vi "Measurement UI.vi"() -> ()   [LabVIEW 2023]
panel:
  out "Measure record dt":dbl
  in  "MeasGraphs":T1(tab)
  out "EfficiencyGraph":T2(graph)
  out "LoadRegulationGraph(V/A)":T3(graph)
  out "LoadRegulationGraph(%)":T3(graph)
  out "OutputCurrentV/STimeGraph":waveform(dbl)(graph) caption="Load Transient"
  in  "Load Current v/s Time":string="LOAD CURRENT vs TIME"
  in  "Output Voltage v/s Time":string="LOAD VOLTAGE vs TIME"
  out "OutputVoltageV/STimeGraph":waveform(dbl)(graph) caption="Load Transient"
  out "Ganged load transient voltages":dbl[](array[numeric])
  out "Ganged load transient currents":dbl[](array[numeric])
  out "Load voltage deviation":dbl[](array[numeric])
  out "Ganged load voltages":dbl[](array[numeric])
  in  "Load current pole-zero ratio":dbl=0.3
  in  "Load current compensation frequency":dbl=180000.0
  in  "Load current gain bandwidth":dbl=14000.0
  in  "Source voltage pole-zero ratio":dbl=2.0
  in  "Source voltage compensation frequency":dbl=3530.0
  in  "Source voltage gain bandwidth":dbl=2000.0
  in  "Load slave resource names":string[](array[string])
  in  "Load master resource name":string
  in  "Source slave resource names":string[](array[string])
  in  "Source master resource name":string
  out "Load sweep points":i32
  out "Source sweep points":i32
  out "Voltage values":dbl[](array[numeric])
  out "Efficiency":dbl[](array[numeric])
  out "Ganged load currents":dbl[](array[numeric])
  in  "MeasConfigurations":T4(tab)=enum."Source Config"
  in  "Measurement timeout":dbl=10.0 caption="MEASUREMENT TIME-OUT" format="%.3ps"
  in  "Nominal output voltage":dbl=1.0 caption="NOMINAL OUTPUT VOLTAGE" format="%.3fV"
  in  "Source delay":dbl=0.005 caption="SOURCE DELAY" format="%.3ps"
  in  "DUT setup time":dbl=1.0 caption="DUT SETUP TIME" format="%.3ps"
  in  "Aperture time":dbl=0.005 caption="APERTURE TIME" format="%.3ps"
  in  "PPSSlaveResourceNames":refnum<k15>[](array[refnum]) caption="SLAVE RESOURCE NAMES"
  in  "PPSMasterResourceName":refnum<k15> caption="MASTER RESOURCE NAME"
  in  "Source stop voltage":dbl=14.0 caption="VOLTAGE STOP LEVEL" format="%#_6pV"
  in  "Source transient response":i32(ring)=1038 caption="TRANSIENT RESPONSE" items=["Slow"=1041, "Normal"=1038, "Fast"=1039, "Custom"=1042]
  in  "Source sense":i32(ring)=1009 caption="SENSE" items=["Local"=1008, "Remote"=1009]
  in  "Source voltage level range":dbl=20.0 caption="VOLTAGE LEVEL RANGE" format="%#_6pV"
  in  "Source start voltage":dbl=6.0 caption="VOLTAGE START LEVEL" format="%#_6pV"
  in  "Source current limit high":dbl=25.0 caption="CURRENT LIMIT/LIMIT HIGH" format="%#_6pA"
  in  "Source current limit range":dbl=25.0 caption="CURRENT LIMIT RANGE" format="%#_6pA"
  in  "Source limit symmetry":enum32{"Symmetric", "Asymmetric"}(ring)=enum."Asymmetric" caption="LIMIT SYMMETRY"
  in  "Source current limit low":dbl=-0.6 caption="CURRENT LIMIT LOW" format="%#_6pA"
  in  "Source system configuration":enum32{"Series", "Parallel"}(ring)=enum."Parallel" caption="SYSTEM CONFIG"
  in  "Source compliance":string="Compliance"
  in  "Source sourceadapt":string="SourceAdapt"
  in  "Source voltage sweep points":i32=4 caption="NO. OF POINTS"
  in  "Source Custom Transient Response":bool
  in  "Load current sweep points/points per decade":i32=10 caption="PTS/PTS PER DECADE"
  in  "Load sweep type":string(combo)="Logarithmic" caption="SWEEP TYPE"
  in  "Load stop current":dbl=50.0 caption="CURRENT STOP LEVEL" format="%#_6pA"
  in  "Load sourceadapt":string="SourceAdapt"
  in  "Load compliance":string="Compliance"
  in  "Load system configuration":enum32{"Series", "Parallel"}(ring)=enum."Parallel" caption="SYSTEM CONFIG"
  in  "Load voltage limit low":dbl caption="VOLTAGE  LIMIT LOW" format="%#_6pV"
  in  "Load limit symmetry":enum32{"Symmetric", "Asymmetric"}(ring) caption="LIMIT SYMMETRY"
  in  "Load voltage limit range":dbl=6.0 caption="VOLTAGE LIMIT RANGE" format="%#_6pV"
  in  "Load voltage limit high":dbl=inf caption="VOLTAGE LIMIT/LIMIT HIGH" format="%#_6p"
  in  "Load start current":dbl=2.0 caption="CURRENT START LEVEL" format="%#_6pA"
  in  "Load current level range":dbl=80.0 caption="CURRENT LEVEL RANGE" format="%#_6pA"
  in  "Load sense":i32(ring)=1009 caption="SENSE" items=["Local"=1008, "Remote"=1009]
  in  "Load transient response":i32(ring)=1038 caption="TRANSIENT RESPONSE" items=["Slow"=1041, "Normal"=1038, "Fast"=1039, "Custom"=1042]
  in  "LoadSlaveResourceNames":refnum<k15>[](array[refnum]) caption="SLAVE RESOURCE NAMES"
  in  "LoadMasterResourceName":refnum<k15> caption="MASTER RESOURCE NAME"
  in  "Load Custom Transient Response":bool
  in  "Sample rate":dbl=0.001 caption="SAMPLE RATE" format="%.3pS/s"
  in  "Level dwell time":dbl=0.001 caption="DWELL TIME" format="%.3ps"
  in  "Enable load transient test?":bool
  in  "Load current falling slew rate":dbl=24.0 caption="CURRENT FALLING SLEW RATE" format="%#_6pA/us"
  in  "Load current rising slew rate":dbl=24.0 caption="CURRENT RISING SLEW RATE" format="%#_6pA/us"
  in  "Load current set point 2":dbl=20.0 caption="CURRENT SET POINT 2" format="%#_6pA"
  in  "Load current set point 1":dbl=1.0 caption="CURRENT SET POINT 1" format="%#_6pA"
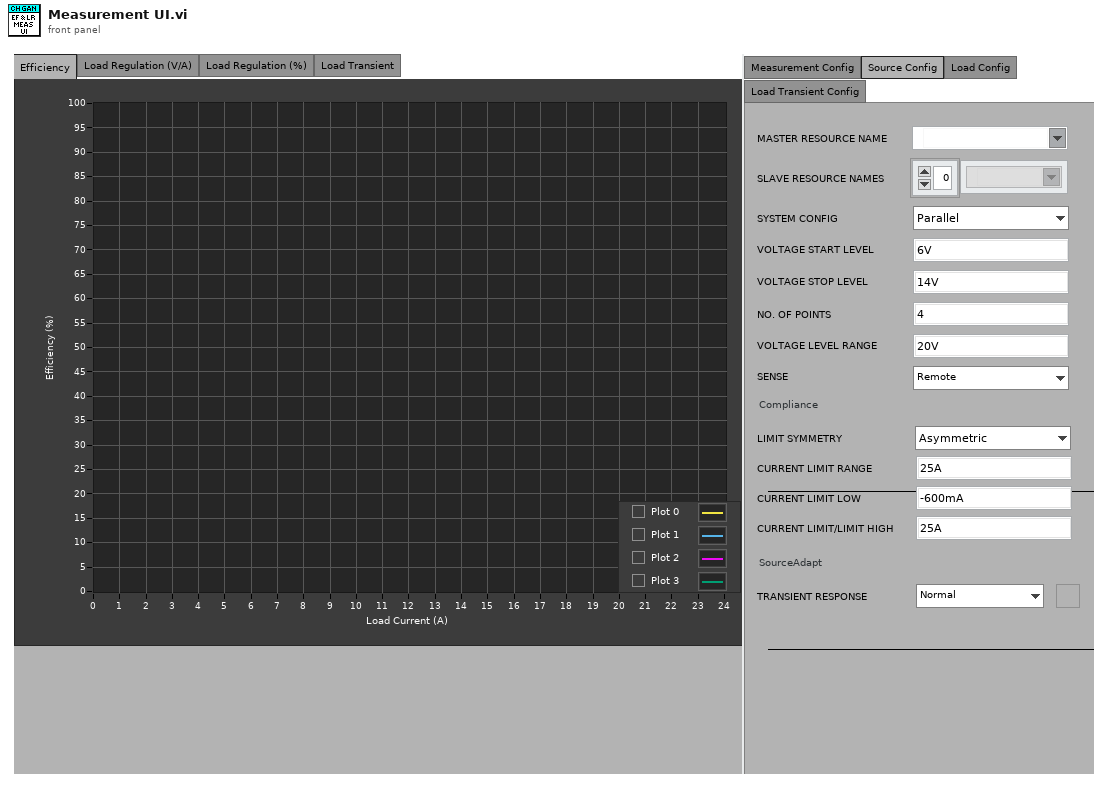
[diagram p1: front panel]
types:
  T1 = enum32{"Efficiency", "Load Regulation (V/A)", "Load Regulation (%)", "Load Transient", "Hidden Controls"}
  T2 = cluster{"Ganged load currents":dbl[], "Efficiency":dbl[]}[]
  T3 = cluster{"Load currents":dbl[], "Efficiency":dbl[]}[]
  T4 = enum32{"Measurement Config", "Source Config", "Load Config", "Load Transient Config"}
  T5 = typedef "SourceAdapt Parameters.ctl" = cluster{"Voltage gain bandwidth":dbl, "Voltage compensation frequency":dbl, "Voltage pole-zero ratio":dbl, "Current gain bandwidth":dbl, "Current compensation frequency":dbl, "Current pole-zero ratio":dbl}
  T6 = cluster{"Ganged load currents":dbl[], "Efficiency":dbl[]}
  T7 = cluster{"Ganged load currents":dbl[], "Ganged load voltages":dbl[]}
  T8 = cluster{"Ganged load currents":dbl[], "Load voltage deviation":dbl[]}
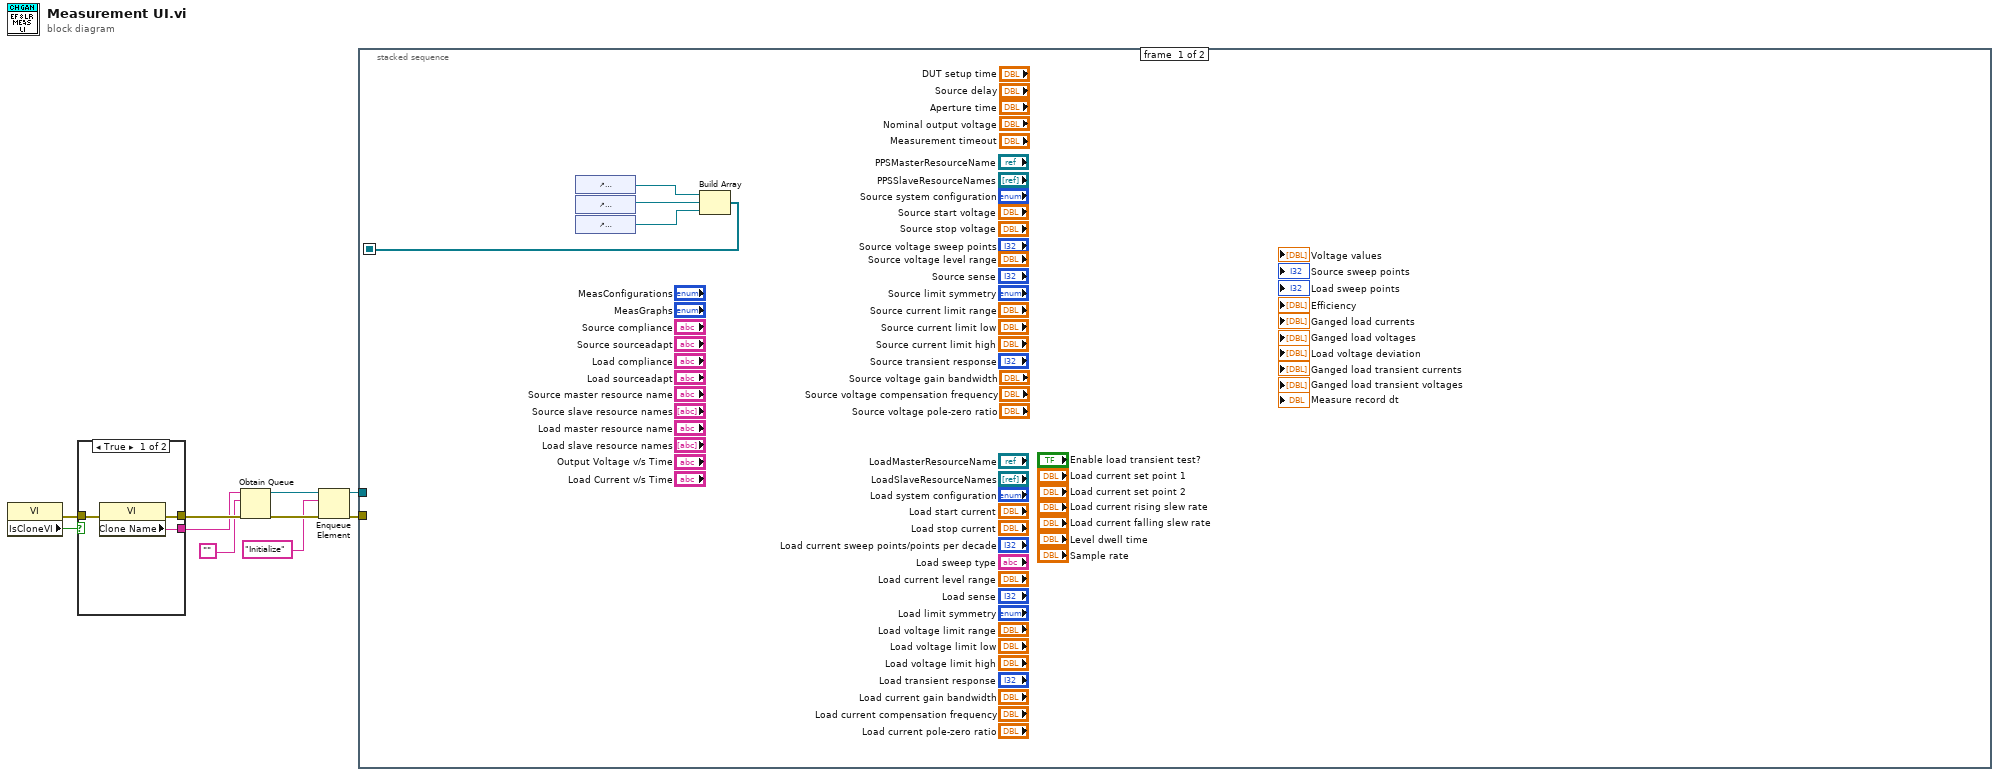
[diagram p0: block diagram]
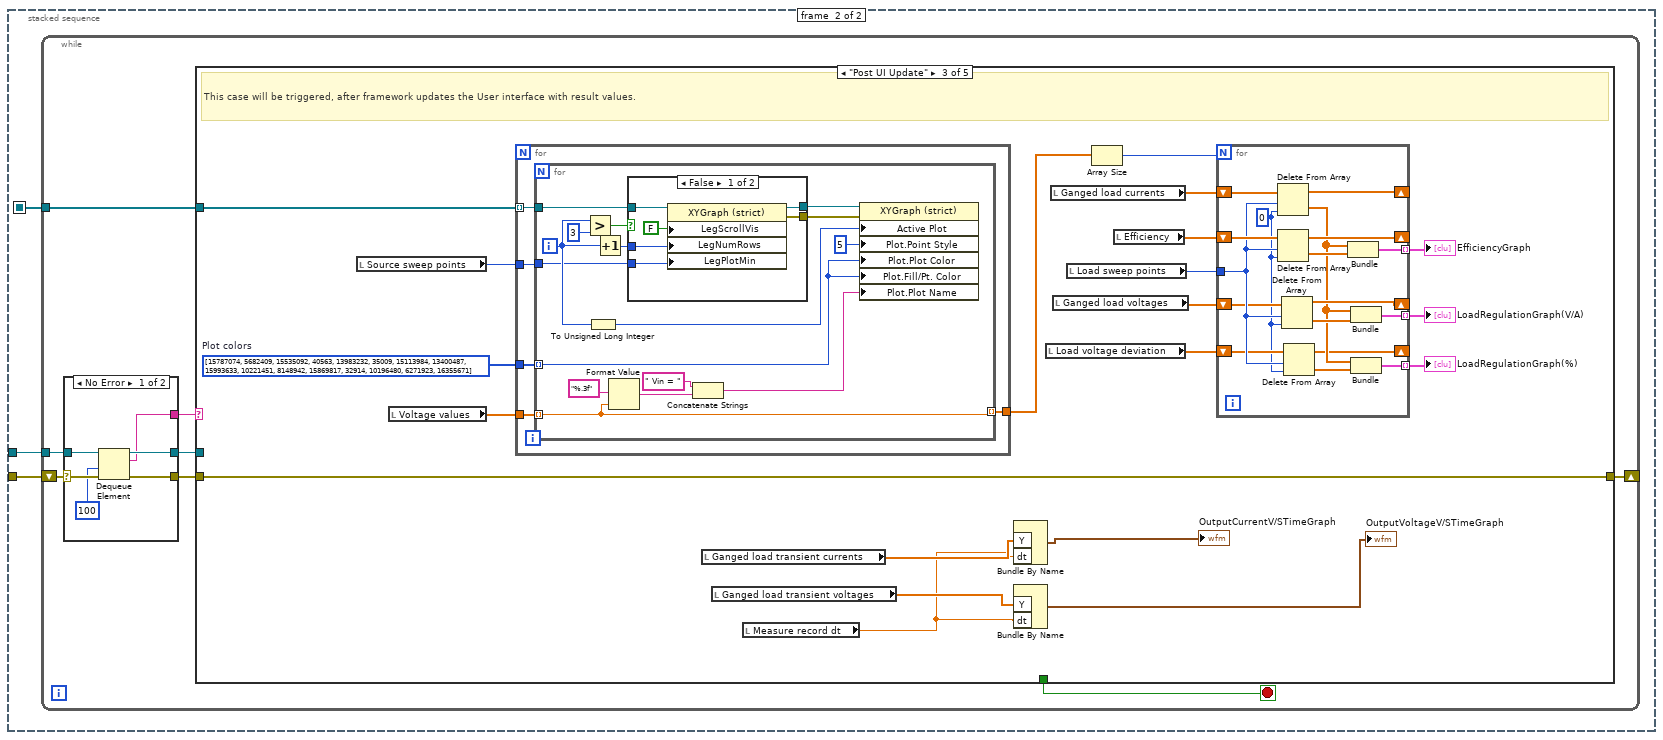
[diagram p2: hidden frame]
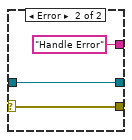
[diagram p3: hidden frame]
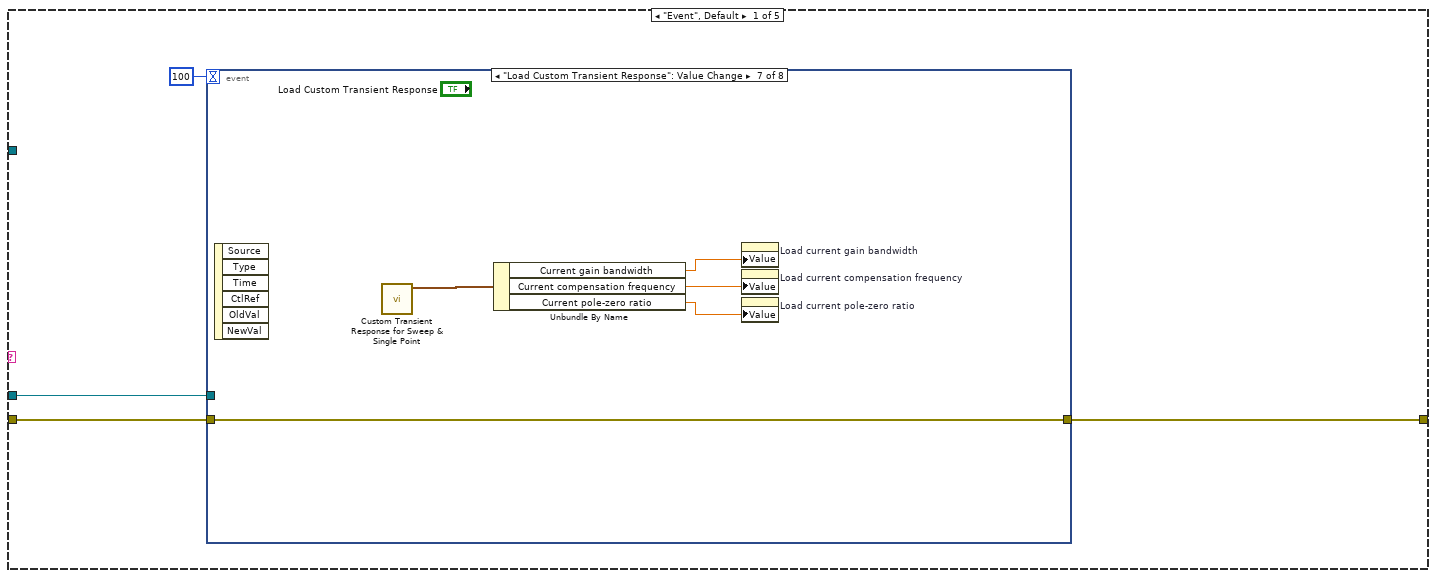
[diagram p4: hidden frame]
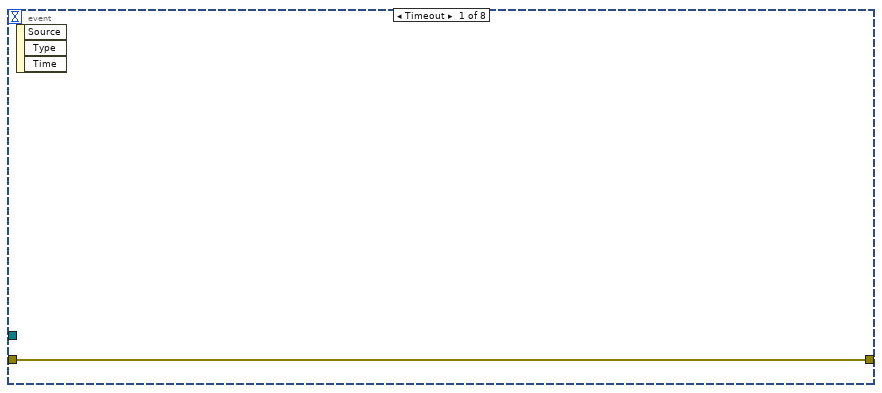
[diagram p5: hidden frame]
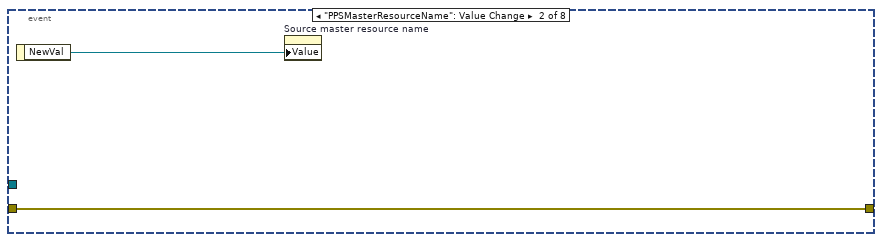
[diagram p6: hidden frame]
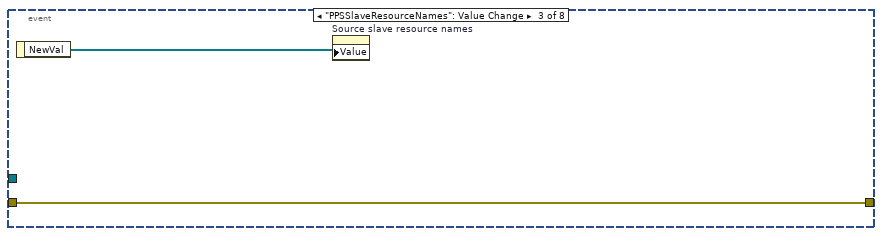
[diagram p7: hidden frame]
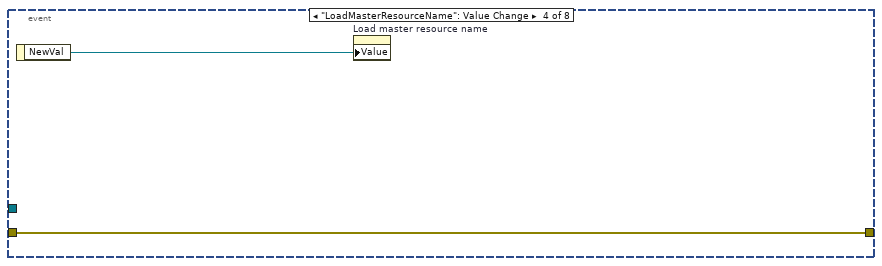
[diagram p8: hidden frame]
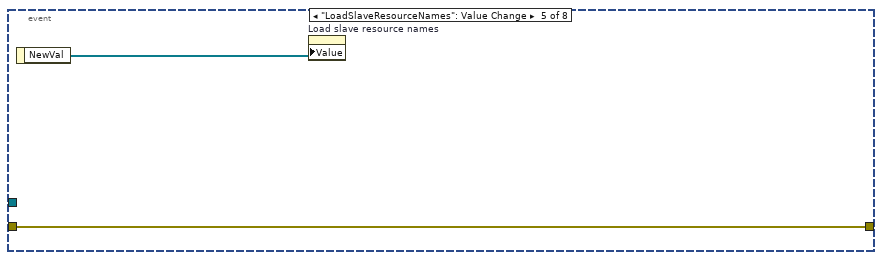
[diagram p9: hidden frame]
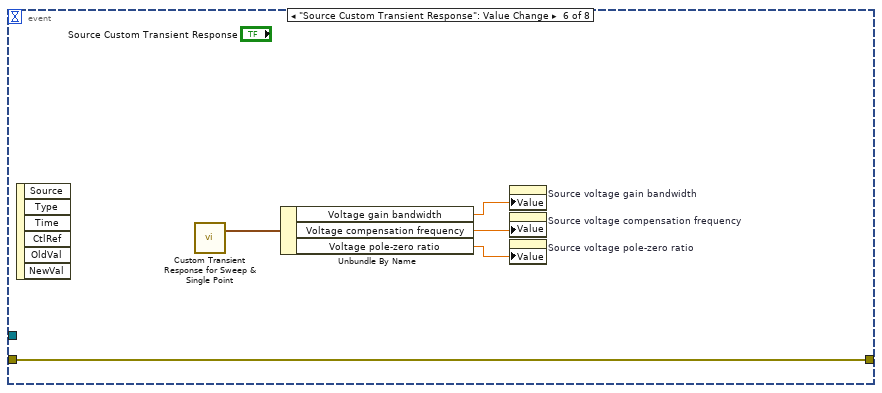
[diagram p10: hidden frame]
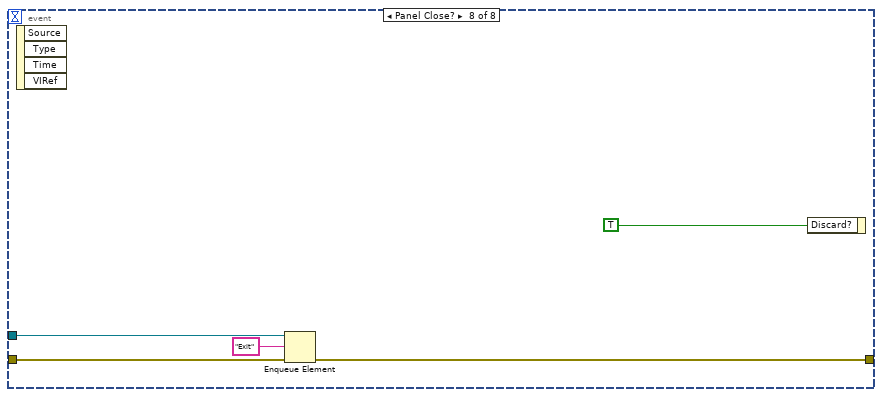
[diagram p11: hidden frame]
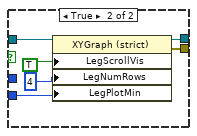
[diagram p13: hidden frame]
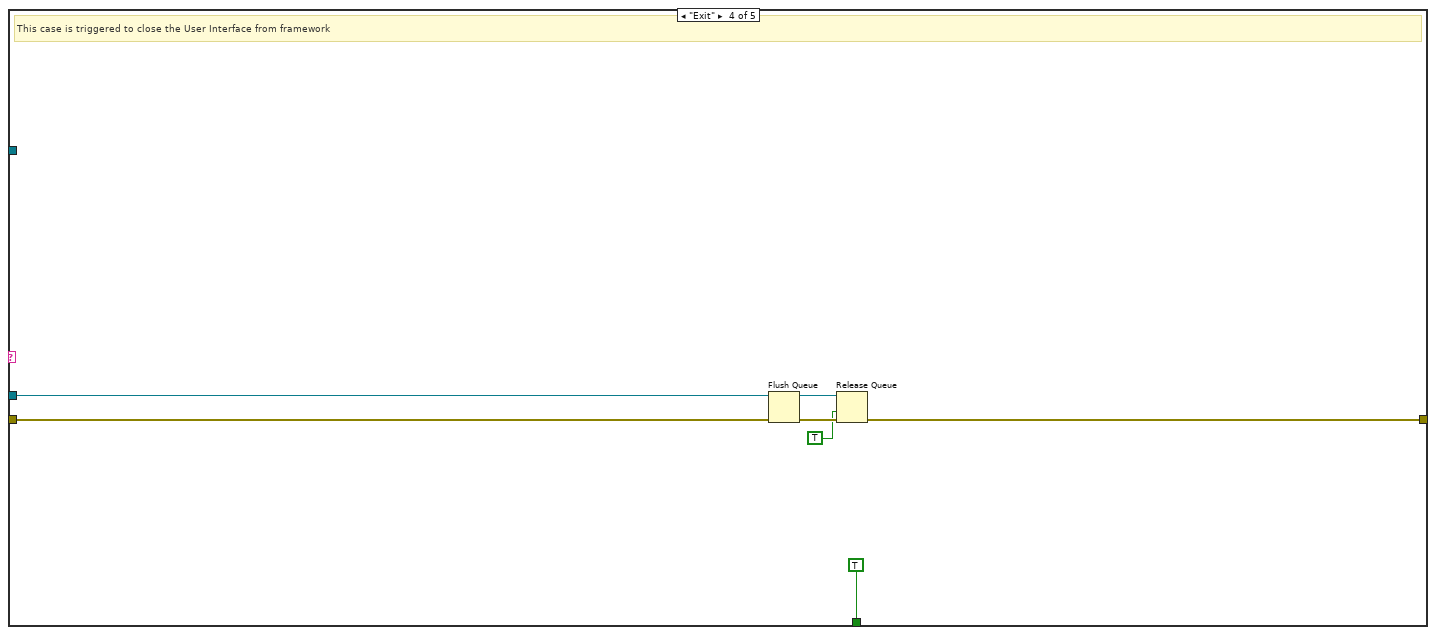
[diagram p14: hidden frame]
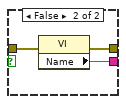
[diagram p16: hidden frame]
diagram:
  n1 = property class="VI"() -> (error out=w1:errorcluster, "IsCloneVI"=w2:bool)  [unwired: 2 in, 1 out]
  n2 = case shown="True" w2 {
    tunnel: [w13 w16] -> w10
    tunnel: [w12 w15] -> w9
    tunnel: w1 -> [w11 w14]
    frame True {
      n3 = property class="VI"(error in=w11) -> (error out=w13:errorcluster, "Clone Name"=w12:string)  [unwired: 1 in, 1 out]
    }
    frame False {
      n4 = property class="VI"(error in=w14) -> (error out=w16:errorcluster, "Name"=w15:string)  [unwired: 1 in, 1 out]
    }
  }
  n5 = Obtain Queue(name (unnamed)=w9, element data type="", error in (no error)=w10) -> (queue out=w6:refnum<queue>, error out=w8:errorcluster)  [unwired: 2 in, 1 out]
  n6 = Enqueue Element(queue=w6, element="Initialize", error in (no error)=w8) -> (queue out=w5:refnum<queue>, error out=w7:errorcluster)  [unwired: 1 in, 1 out]
  n7 = stacked-sequence {
    seq-local: [w17 _] -> [_ w21]
    tunnel: w7 -> [_ w23]
    tunnel: w5 -> [_ w22]
    frame #0 {
      n8 = control-ref of="EfficiencyGraph"() -> (w20:refnum<vi>)
      n9 = control-ref of="LoadRegulationGraph(V/A)"() -> (w19:refnum<vi>)
      n10 = control-ref of="LoadRegulationGraph(%)"() -> (w18:refnum<vi>)
      n11 = Build Array(w20, w19, w18) -> (w17:refnum<vi>[])
    }
    frame #1 {
      n12 = while {
        shift-right: [w26] -> _
        shift-left: w23 -> [w31]
        tunnel: w22 -> [w29]
        tunnel: w21 -> [w24]
        stop <- w25 stop-if-true
        n13 = case shown="No Error" w31 {
          selector: w31 -> [w37 w40]
          tunnel: [w36 w40] -> w30
          tunnel: w29 -> [w35 w39]
          tunnel: [w34 w39] -> w28
          tunnel: [w33 "Handle Error"] -> w27
          frame No Error {
            n14 = Dequeue Element(queue=w35, timeout in ms (-1)=100, error in (no error)=w37) -> (queue out=w34:refnum<queue>, element=w33:string, error out=w36:errorcluster)  [unwired: 1 out]
          }
          frame Error {
          }
        }
        n15 = case shown="\"Post UI Update\"" w27 {
          tunnel: w30 -> [w43 w69 w89 w146 w147]
          tunnel: w28 -> [w41 _ _ w144 _]
          tunnel: [w44 w69 w89 w141 w147] -> w26
          tunnel: [_ _ _ TRUE _] -> w25
          tunnel: w24 -> [_ _ w77 _ _]
          frame "Event", Default {
            n16 = event shown="[6] \"Load Custom Transient Response\": Value Change" {
              selector: _ -> [_ _ _ _ _ _ _ _]
              dyn-events: _ -> [_ _ _ _ _ _ _ _]
              timeout: 100 -> [_ _ _ _ _ _ _ _]
              tunnel: [w45 w47 w49 w50 w52 w57 w62 w66] -> w44
              tunnel: w43 -> [w45 w47 w49 w50 w52 w57 w62 w67]
              tunnel: w41 -> [_ _ _ _ _ _ _ w65]
              event Timeout {
                n17 = event-data() -> ()  [unwired: 1 in, 3 out]
              }
              event "PPSMasterResourceName": Value Change {
                n18 = event-data() -> ("NewVal"=w46:refnum<k15>)  [unwired: 1 in]
                n19 = property on="Source master resource name" class="Str"("Value"=w46) -> ()  [unwired: 2 in, 2 out]
              }
              event "PPSSlaveResourceNames": Value Change {
                n20 = event-data() -> ("NewVal"=w48:refnum<k15>[])  [unwired: 1 in]
                n21 = property on="Source slave resource names" class="Arr (strict)"("Value"=w48) -> ()  [unwired: 2 in, 2 out]
              }
              event "LoadMasterResourceName": Value Change {
                n22 = event-data() -> ("NewVal"=w51:refnum<k15>)  [unwired: 1 in]
                n23 = property on="Load master resource name" class="Str"("Value"=w51) -> ()  [unwired: 2 in, 2 out]
              }
              event "LoadSlaveResourceNames": Value Change {
                n24 = event-data() -> ("NewVal"=w53:refnum<k15>[])  [unwired: 1 in]
                n25 = property on="Load slave resource names" class="Arr (strict)"("Value"=w53) -> ()  [unwired: 2 in, 2 out]
              }
              event "Source Custom Transient Response": Value Change {
                n26 = event-data() -> ()  [unwired: 1 in, 6 out]
                n27 = call "Custom Transient Response for Sweep & Single Point.vi"() -> ("SourceAdapt Parameters"=w58:T5)  [unwired: 11 in]
                n28 = Unbundle By Name(w58) -> ("Voltage gain bandwidth"=w55:dbl, "Voltage compensation frequency"=w56:dbl, "Voltage pole-zero ratio"=w54:dbl)
                n29 = property on="Source voltage gain bandwidth" class="DigNum (strict)"("Value"=w55) -> ()  [unwired: 2 in, 2 out]
                n30 = property on="Source voltage compensation frequency" class="DigNum (strict)"("Value"=w56) -> ()  [unwired: 2 in, 2 out]
                n31 = property on="Source voltage pole-zero ratio" class="DigNum (strict)"("Value"=w54) -> ()  [unwired: 2 in, 2 out]
              }
              event "Load Custom Transient Response": Value Change {
                n32 = event-data() -> ()  [unwired: 1 in, 6 out]
                n33 = call "Custom Transient Response for Sweep & Single Point.vi"() -> ("SourceAdapt Parameters"=w63:T5)  [unwired: 11 in]
                n34 = Unbundle By Name(w63) -> ("Current gain bandwidth"=w59:dbl, "Current compensation frequency"=w61:dbl, "Current pole-zero ratio"=w60:dbl)
                n35 = property on="Load current gain bandwidth" class="DigNum (strict)"("Value"=w59) -> ()  [unwired: 2 in, 2 out]
                n36 = property on="Load current compensation frequency" class="DigNum (strict)"("Value"=w61) -> ()  [unwired: 2 in, 2 out]
                n37 = property on="Load current pole-zero ratio" class="DigNum (strict)"("Value"=w60) -> ()  [unwired: 2 in, 2 out]
              }
              event Panel Close? {
                n38 = event-data() -> ()  [unwired: 1 in, 4 out]
                n39 = Enqueue Element(queue=w65, element="Exit", error in (no error)=w67) -> (error out=w66:errorcluster)  [unwired: 1 in, 2 out]
                n40 = event-data("Discard?"=TRUE) -> ()  [unwired: 1 in, 1 out]
              }
            }
          }
          frame "Initialize" {
          }
          frame "Post UI Update" {
            w84 = u32[] [15787074, 5682409, 15535092, 40563, 13983232, 35009, 15113984, 13400487, 15993633, 10221451, 8148942, 15869817, 32914, 10196480, 6271923, 16355671]  # Plot colors
            # "This case will be triggered, after framework updates the User interface with result values."
            n41 = local read "Source sweep points"() -> (w82:i32)
            n42 = local read "Voltage values"() -> (w83:dbl[])
            n43 = for {
              tunnel: w84 -> [w94]
              tunnel: w77 -> [w93] mode=indexing
              tunnel: w83 -> [w92]
              tunnel: w82 -> [w91]
              tunnel: [w90] -> w76
              n44 = for {
                tunnel: w92 -> [w107] mode=indexing
                tunnel: [w107] -> w90 mode=indexing
                tunnel: w93 -> [w100]
                tunnel: w91 -> [w97]
                tunnel: w94 -> [w103] mode=indexing
                i -> [w101]
                n45 = Greater?(x=w101, y=3) -> (0:w105:bool)
                n46 = To Unsigned Long Integer(number=w101) -> (unsigned 32bit integer=w104:u32)
                n47 = Increment(x=w101) -> (x+1=w99:i32)
                n48 = Format Value(format string="%.3f", value (0)=w107) -> (output string=w110:string)  [unwired: 1 out]
                n49 = case shown="False" w105 {
                  tunnel: w100 -> [w116 w122]
                  tunnel: w99 -> [w115 _]
                  tunnel: [w114 w121] -> w98
                  tunnel: w97 -> [w112 w117]
                  tunnel: [w113 w120] -> w96
                  frame False {
                    n50 = property on="Property Node" class="XYGraph (strict)"(reference=w116, "LegScrollVis"=FALSE ("Legend:Scrollbar Visible"), "LegNumRows"=w115, "LegPlotMin"=w112) -> (reference out=w114:refnum<vi>, error out=w113:errorcluster)  [unwired: 1 in]
                  }
                  frame True {
                    n51 = property on="Property Node" class="XYGraph (strict)"(reference=w122, "LegScrollVis"=TRUE ("Legend:Scrollbar Visible"), "LegNumRows"=u32 4 ("Legend:Number of Rows"), "LegPlotMin"=w117) -> (reference out=w121:refnum<vi>, error out=w120:errorcluster)  [unwired: 1 in]
                  }
                }
                n52 = Concatenate Strings(" Vin = " ("string"), w110) -> (w95:string)
                n53 = property on="Property Node" class="XYGraph (strict)"(reference=w98, error in=w96, "Active Plot"=w104, "Plot.Point Style"=u8 5, "Plot.Plot Color"=w103, "Plot.Fill/Pt. Color"=w103, "Plot.Plot Name"=w95) -> ()  [unwired: 2 out]
              }
            }
            n54 = local read "Ganged load transient currents"() -> (w71:dbl[])
            n55 = local read "Ganged load transient voltages"() -> (w72:dbl[])
            n56 = local read "Measure record dt"() -> (w70:dbl)
            n57 = Bundle By Name("Y"=w71, "dt"=w70) -> (→"OutputCurrentV/STimeGraph":waveform(dbl))  [unwired: 1 in]
            n58 = Bundle By Name("Y"=w72, "dt"=w70) -> (→"OutputVoltageV/STimeGraph":waveform(dbl))  [unwired: 1 in]
            n59 = local read "Load voltage deviation"() -> (w80:dbl[])
            n60 = local read "Ganged load currents"() -> (w88:dbl[])
            n61 = local read "Ganged load voltages"() -> (w81:dbl[])
            n62 = local read "Load sweep points"() -> (w85:i32)
            n63 = Array Size(array=w76) -> (size(s)=w75:i32)
            n64 = local read "Efficiency"() -> (w87:dbl[])
            n65 = for {
              N: w75 -> [_]
              tunnel: [w139] -> w86 mode=indexing
              shift-right: [w138] -> _
              shift-left: w88 -> [w136]
              shift-right: [w134] -> _
              shift-left: w87 -> [w135]
              tunnel: w85 -> [w133]
              shift-right: [w130] -> _
              shift-left: w81 -> [w132]
              shift-right: [w127] -> _
              shift-left: w80 -> [w131]
              tunnel: [w126] -> w78 mode=indexing
              tunnel: [w125] -> w79 mode=indexing
              w124 = 0 ("index")
              n66 = Delete From Array(array=w136, length=w133, index=w124) -> (deleted portion=w128:dbl[], array with subset deleted=w138:dbl[])
              n67 = Delete From Array(array=w135, length=w133, index=w124) -> (deleted portion=w137:dbl[], array with subset deleted=w134:dbl[])
              n68 = Delete From Array(array=w132, length=w133, index=w124) -> (deleted portion=w129:dbl[], array with subset deleted=w130:dbl[])
              n69 = Delete From Array(array=w131, length=w133, index=w124) -> (deleted portion=w123:dbl[], array with subset deleted=w127:dbl[])
              n70 = Bundle("Ganged load currents"=w128, "Efficiency"=w137) -> (w139:T6)  [unwired: 1 in]
              n71 = Bundle("Ganged load currents"=w128, "Ganged load voltages"=w129) -> (w125:T7)  [unwired: 1 in]
              n72 = Bundle("Ganged load currents"=w128, "Load voltage deviation"=w123) -> (w126:T8)  [unwired: 1 in]
            }
            "EfficiencyGraph" <- w86
            "LoadRegulationGraph(V/A)" <- w79
            "LoadRegulationGraph(%)" <- w78
          }
          frame "Exit" {
            # "This case is triggered to close the User Interface from framework"
            n73 = Flush Queue(queue=w144, error in (no error)=w146) -> (queue out=w143:refnum<queue>, error out=w142:errorcluster)  [unwired: 1 out]
            n74 = Release Queue(queue=w143, force destroy? (F)=TRUE, error in (no error)=w142) -> (error out=w141:errorcluster)  [unwired: 2 out]
          }
          frame "Handle Error" {
          }
        }
      }
    }
  }
